vi "CIET Data Write Only Client Dummy.vi"() -> ()   [LabVIEW 2017]
uses:
  <vilib>/OPCUA/controls/Write Status.ctl
  <vilib>/OPCUA/controls/NodeId.ctl
  <vilib>/OPCUA/client/Multiple Write Double Array.vi
  <vilib>/OPCUA/NI OPC UA Client.lvlib
panel:
  in  "element":dbl
  in  "array 3":dbl[](array[numeric])
  in  "array 2":dbl[](array[numeric])
  in  "array":dbl
  in  "Stop Broadcasting":bool
  out "Send Loop":i32
  in  "Time Stamp":timestamp
  in  "Node Status":T1 items=["Good"=0, "Uncertain_InitialValue"=1083310080, "Uncertain_LastUsableValue"=1083179008, "Uncertain_SensorNotAccurate"=1083375616, "Uncertain_EngineeringUnitsExceeded"=1083441152, "Bad_NoCommunication"=2150694912, "Bad_NotReadable"=2151284736, "Bad_NotWritable"=2151350272, "Bad_OutOfRange"=2151415808, "Bad_WaitingForInitialData"=2150760448]
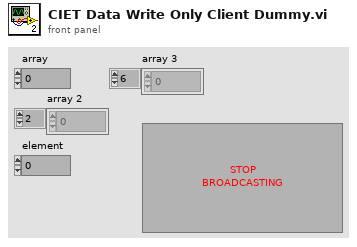
[diagram p1: front panel]
types:
  T1 = typedef "Write Status.ctl" = u32
  T2 = typedef "OPC UA Client Refnum.ctl" = refnum<k21>
  T3 = typedef "NodeId.ctl" = string
  T4 = cluster{"node ID":T3, "value":dbl[], "timestamp (current time)":timestamp, "node status":T1}
  T5 = cluster{"node ID":T3, "value":dbl[], "timestamp (current time)":timestamp, "node status":T1}[]
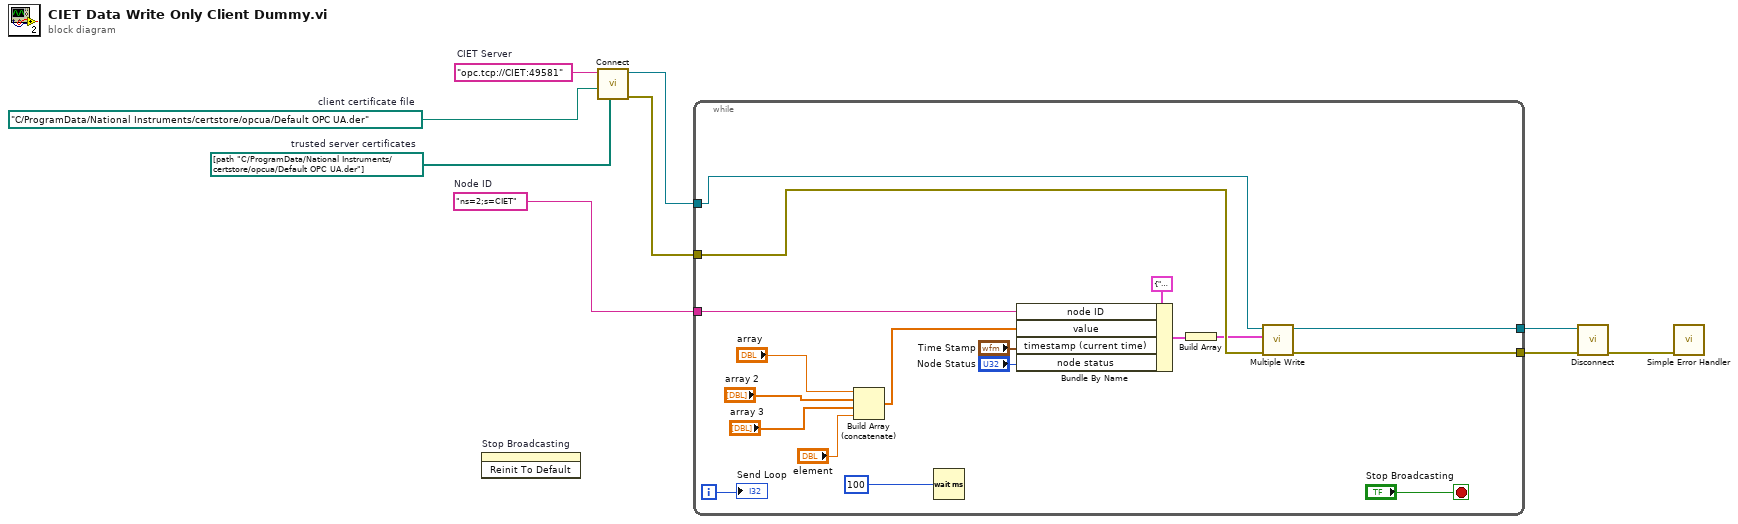
[diagram p0: block diagram]
diagram:
  w1 = path[] [path "C:/ProgramData/National Instruments/certstore/opcua/Default OPC UA.der"]  # trusted server certificates
  w2 = path "C:/ProgramData/National Instruments/certstore/opcua/Default OPC UA.der"  # client certificate file
  w5 = "ns=2;s=CIET"  # Node ID
  w8 = "opc.tcp://CIET:49581"  # CIET Server
  n1 = invoke on="Stop Broadcasting" class="Bool (strict)" method="Reinit To Default"() -> ()  [unwired: 3 in, 3 out]
  n2 = call <vilib>:"Connect.vi"("trusted server certificates"=w1, "client certificate file"=w2, "server endpoint URL"=w8) -> ("error out"=w7:errorcluster, "OPC UA client refnum out"=w6:T2)  [unwired: 6 in, 1 out]
  n3 = while {
    tunnel: w5 -> [w25]
    tunnel: w6 -> [w22]
    tunnel: w7 -> [w21]
    tunnel: [w24] -> w4
    tunnel: [w23] -> w3
    i -> [w26]
    stop <- "Stop Broadcasting" stop-if-true
    n4 = Build Array (concatenate)("array", "array 2", "array 3", "element") -> (w17:dbl[])
    n5 = Wait (ms)(milliseconds to wait=u32 100) -> ()  [unwired: 1 out]
    n6 = Bundle By Name(cluster=T4 {"node ID"="", "value"=[], "timestamp (current time)"=timestamp(0 s since 1904-01-01), "node status"=0} ("request"), "node ID"=w25, "value"=w17, "timestamp (current time)"="Time Stamp", "node status"="Node Status") -> (w15:T4)
    n7 = Build Array(w15) -> (w14:T5)
    n8 = call-poly <vilib>:"Multiple Write.vi"("error in (no error)"=w21, "requests"=w14, "OPC UA client refnum in"=w22) -> ("error out"=w23:errorcluster, "OPC UA client refnum out"=w24:T2)  [unwired: 5 in, 2 out]
    "Send Loop" <- w26
  }
  n9 = call <vilib>:"Disconnect.vi"("error in (no error)"=w3, "OPC UA client refnum in"=w4) -> ("error out"=w9:errorcluster)  [unwired: 9 in]
  n10 = call <vilib>:"Simple Error Handler.vi"("error in (no error)"=w9) -> ()  [unwired: 4 in, 5 out]
